vi "Autonomous Independent.vi"() -> ()   [LabVIEW 2018]
doc: "This VI is called when autonomous begins, and will automatically be terminated when autonomous ends. You can carry out timed or sensor driven robot movement independently without needing to return to the caller."
uses:
  <vilib>/Rock Robotics/WPI/ThirdParty/Phoenix-LabVIEW/Motor Controller/Controls/CTRE_Phoenix_MotorControl_ControlMode.ctl
  <vilib>/Rock Robotics/WPI/Utilities/WPI_GetSetVariantRefNum.vi
  <vilib>/Rock Robotics/Network Tables/NT Read String.vi
  <vilib>/Rock Robotics/Network Tables/NT Write Numeric Array.vi
  <vilib>/Rock Robotics/WPI/ThirdParty/Phoenix-LabVIEW/Motor Controller/Get/CTRE_Phoenix_MotorController_GetOutputCurrent_Enhanced.vi
  <vilib>/Rock Robotics/WPI/ThirdParty/Phoenix-LabVIEW/Motor Controller/Get/CTRE_Phoenix_MotorController_GetSelectedSensorData.vi
  <vilib>/Rock Robotics/WPI/RobotDrive/WPI_RobotDriveArcadeDrive_Standard(NoSaturation).vi
panel:
  out "Current Left":T1(graph)
  out "Current Right":T1(graph)
  out "Velocity":T2(graph)
  out "Position":T3(graph)
  in  "Speed %":dbl=0.4
  in  "Array of robot movements":T4(array[cluster])=[{"X Joystick Value"=0.39393939393939403, "Y Joystick Value"=0.0, "Delay (sec)"=1.0, "Movement Name"="turn"}, {"X Joystick Value"=-0.3737373737373737, "Y Joystick Value"=0.0, "Delay (sec)"=1.0, "Movement Name"="turn back"}] {"Y Joystick Value" scale=1.0..-1.0; "X Joystick Value" scale=-1.0..1.0}
  # "Be sure to right-click and choose Data Operations>>Make Current Value default if you want to save the array values with the VI"
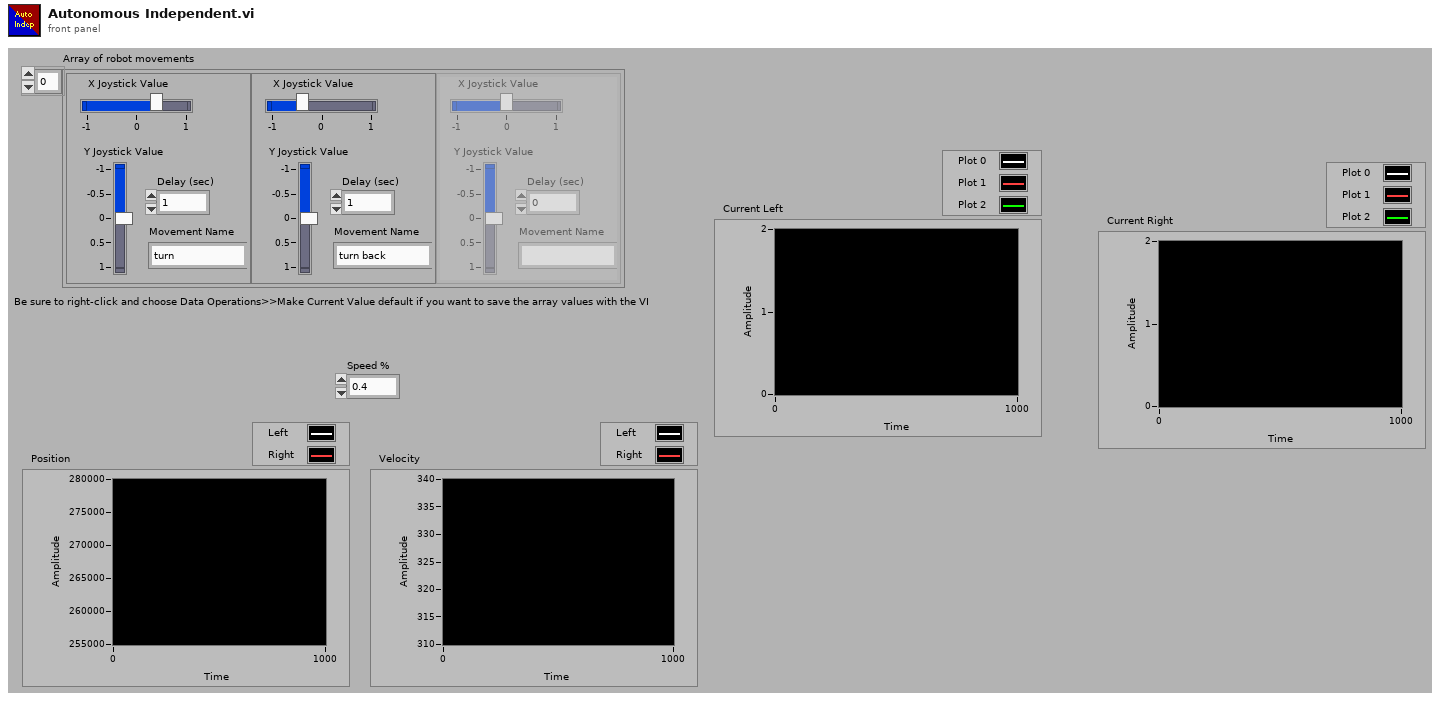
[diagram p1: front panel]
types:
  T1 = cluster{"Output Current":dbl, "Output Current":dbl, "Output Current":dbl}
  T2 = cluster{"Velocity (Raw Sensor Units per 100 ms)":i32, "Velocity (Raw Sensor Units per 100 ms)":i32}
  T3 = cluster{"Position (Raw Sensor Units)":i32, "Position (Raw Sensor Units)":i32}
  T4 = cluster{"X Joystick Value":dbl, "Y Joystick Value":dbl, "Delay (sec)":dbl, "Movement Name":string}[]
  T5 = typedef "WPI_JoystickDevRef.ctl" = cluster{"Device":T6}
  T6 = typedef "WPI_JoystickDeviceEnum.ctl" = enum16{"USB 0", "USB 1", "USB 2", "USB 3", "USB 4", "USB 5"}
  T7 = typedef "WPI_MotorControlDeviceRef.ctl" = cluster{"DeviceStatus":errorcluster, "Type":T8, "PWM":cluster{"PWM Channel":T9, "DeadBand":T10}, "CAN":cluster{"Device Number":u8, "SetOutput VI Ref":variant, "GetOutput VI Ref":variant, "Enable VI Ref":variant, "Disable VI Ref":variant, "Data":variant}, "Invert":bool, "DIO PWM":cluster{"PWM \"Enable\" Channel":T9, "DIOChannel":T11, "PWM Rate":dbl}}
  T8 = typedef "WPI_MotorControlType.ctl" = enum16{"PWM", "CAN", "DIO PWM"}
  T9 = typedef "FPGA_DIOPWMChannel.ctl" = enum8{"PWM 0", "PWM 1", "PWM 2", "PWM 3", "PWM 4", "PWM 5", "PWM 6", "PWM 7", "PWM 8", "PWM 9", "PWM MXP 0", "PWM MXP 1", "PWM MXP 2", "PWM MXP 3", "PWM MXP 4", "PWM MXP 5", "PWM MXP 6", "PWM MXP 7", "PWM MXP 8", "PWM MXP 9", "Invalid"}
  T10 = typedef "WPI_PWMDeadband.ctl" = cluster{"Name":string, "maxPositivePwm":i32, "minPositivePwm":i32, "centerPwm":i32, "maxNegativePwm":i32, "minNegativePwm":i32, "angularRange":u16}
  T11 = typedef "FPGA_DIOChannel.ctl" = enum8{"DIO 0", "DIO 1", "DIO 2", "DIO 3", "DIO 4", "DIO 5", "DIO 6", "DIO 7", "DIO 8", "DIO 9", "DIO MXP 0", "DIO MXP 1", "DIO MXP 2", "DIO MXP 3", "DIO MXP 4", "DIO MXP 5", "DIO MXP 6", "DIO MXP 7", "DIO MXP 8", "DIO MXP 9", "DIO MXP 10", "DIO MXP 11", "DIO MXP 12", "DIO MXP 13", "DIO MXP 14", "DIO MXP 15", "SPI Port CS1", "SPI Port CS2", "SPI Port CS3", "SPI Port MISO", "SPI Port MOSI", "Invalid"}
  T12 = typedef "CTRE_Phoenix_MotorControl_ControlMode.ctl" = u16
  T13 = typedef "WPI_RobotDriveDevRef.ctl" = cluster{"DevStatus":errorcluster, "Motors[]":T7[], "Square Inputs":bool, "Max Output":dbl}
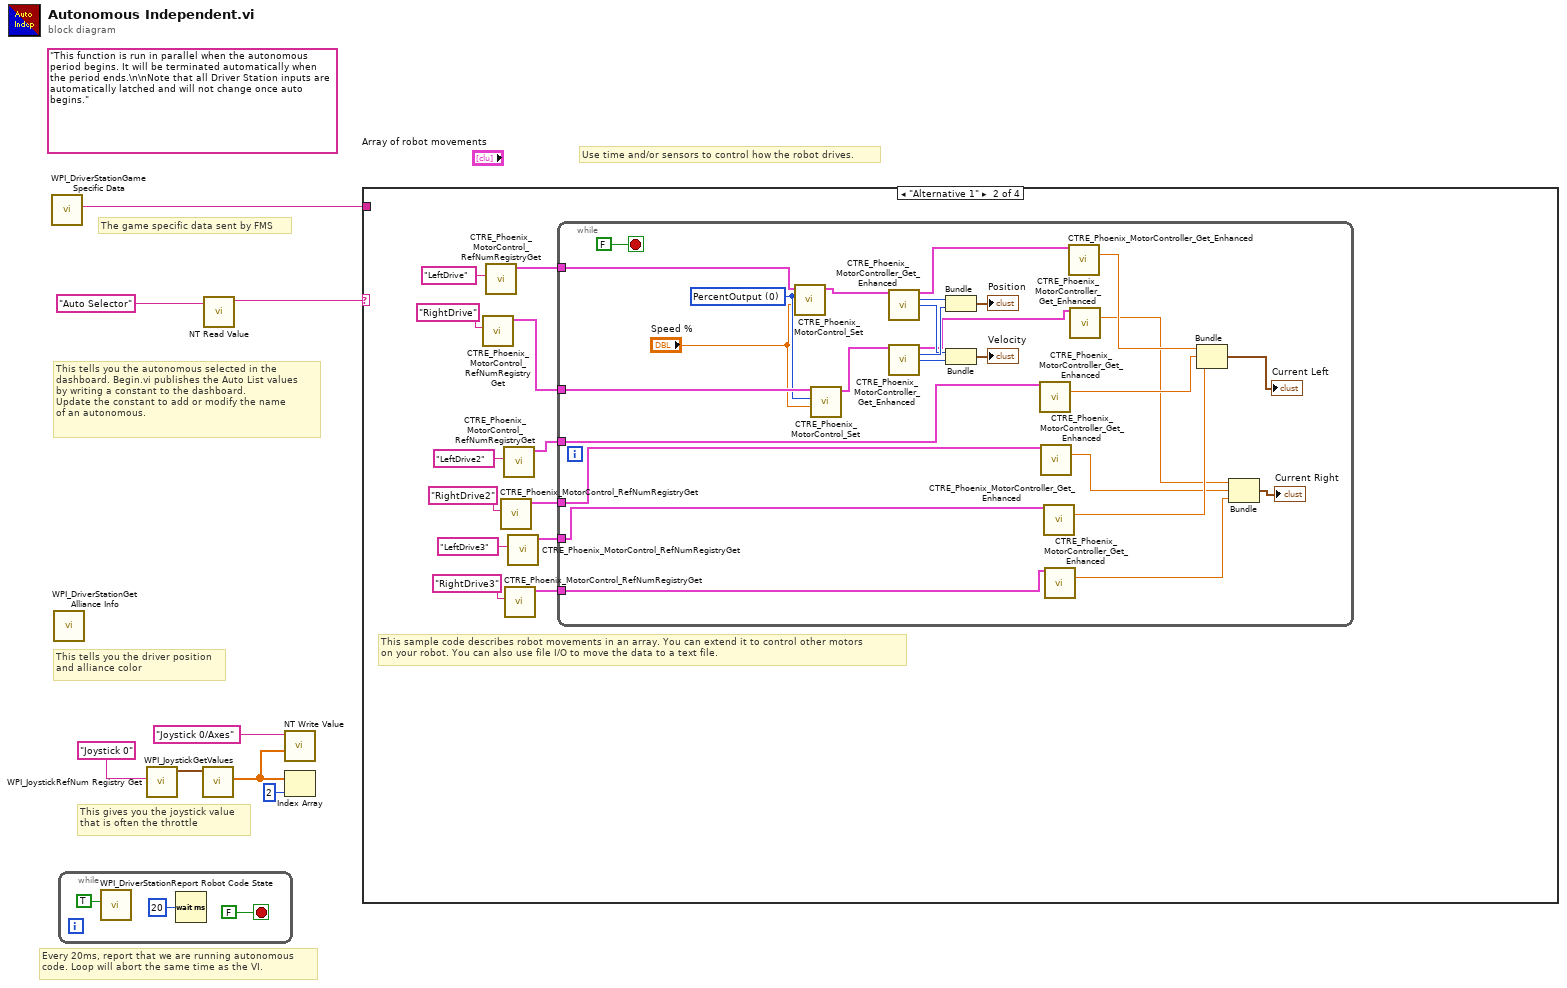
[diagram p0: block diagram]
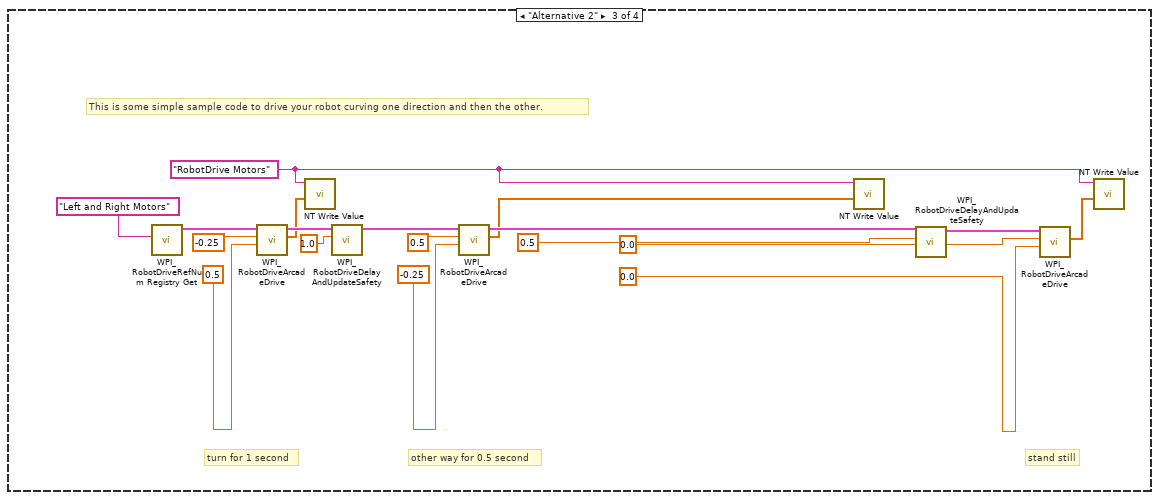
[diagram p3: hidden frame]
diagram:
  (unwired) "This function is run in parallel when the autonomous period begins. It will be terminated automatically when the period ends.\n\nNote that all Driver Station inputs are automatically latched and will not change once auto begins."
  # "The game specific data sent by FMS"
  # "This tells you the autonomous selected in the \ndashboard. Begin.vi publishes the Auto List values\nby writing a constant to the dashboard.\nUpdate the constant to add or modify the name\nof an autonomous."
  # "Every 20ms, report that we are running autonomous\ncode. Loop will abort the same time as the VI."
  # "This gives you the joystick value\nthat is often the throttle"
  # "Use time and/or sensors to control how the robot drives."
  # "This tells you the driver position\nand alliance color"
  n1 = call <vilib>:"WPI_DriverStationGame Specific Data.vi"() -> ("Game Specific Data"=w1:string)  [unwired: 11 in]
  n2 = call <vilib>:"WPI_DriverStationGet Alliance Info.vi"() -> ()  [unwired: 12 out]
  n3 = while {
    stop <- FALSE stop-if-true
    n4 = call <vilib>:"WPI_DriverStationReport Robot Code State.vi"("Autonomous"=TRUE) -> ()  [unwired: 10 in, 1 out]
    n5 = Wait (ms)(milliseconds to wait=u32 20) -> ()  [unwired: 1 out]
  }
  n6 = call <vilib>:"WPI_JoystickRefNum Registry Get.vi"("refnum name"="Joystick 0") -> ("JoystickDevRef"=w7:T5)  [unwired: 1 in, 9 out]
  n7 = call <vilib>:"WPI_JoystickGetValues.vi"("JoystickDevRef"=w7) -> ("Axes"=w3:dbl[])  [unwired: 6 in, 4 out]
  n8 = call-poly <vilib>:"NT Read Value.vi"("Name"="Auto Selector") -> ("String"=w4:string)  [unwired: 9 in, 1 out]
  n9 = call-poly <vilib>:"NT Write Value.vi"("Numeric Array"=w3, "Name"="Joystick 0/Axes") -> ()  [unwired: 9 in, 1 out]
  n10 = Index Array(array=w3, index=2) -> ()  [unwired: 1 out]
  n11 = case shown="\"Alternative 1\"" w4 {
    tunnel: w1 -> [_ _ _ _]
    frame Default {
      # "You can put your main auto here, or you can right-click on the case and make any\nother frame be the default case."
      # "This is the frame that will execute if no selection is made, or if it is not recognized"
    }
    frame "Alternative 1" {
      # "This sample code describes robot movements in an array. You can extend it to control other motors\non your robot. You can also use file I/O to move the data to a text file."
      n12 = call <vilib>:"CTRE_Phoenix_MotorControl_RefNumRegistryGet.vi"("refnum name"="RightDrive") -> ("PhoenixMotorControlDevRef"=w20:T7)  [unwired: 9 in, 1 out]
      n13 = call <vilib>:"CTRE_Phoenix_MotorControl_RefNumRegistryGet.vi"("refnum name"="LeftDrive") -> ("PhoenixMotorControlDevRef"=w21:T7)  [unwired: 9 in, 1 out]
      n14 = call <vilib>:"CTRE_Phoenix_MotorControl_RefNumRegistryGet.vi"("refnum name"="RightDrive2") -> ("PhoenixMotorControlDevRef"=w14:T7)  [unwired: 9 in, 1 out]
      n15 = call <vilib>:"CTRE_Phoenix_MotorControl_RefNumRegistryGet.vi"("refnum name"="LeftDrive2") -> ("PhoenixMotorControlDevRef"=w15:T7)  [unwired: 9 in, 1 out]
      n16 = call <vilib>:"CTRE_Phoenix_MotorControl_RefNumRegistryGet.vi"("refnum name"="RightDrive3") -> ("PhoenixMotorControlDevRef"=w12:T7)  [unwired: 9 in, 1 out]
      n17 = call <vilib>:"CTRE_Phoenix_MotorControl_RefNumRegistryGet.vi"("refnum name"="LeftDrive3") -> ("PhoenixMotorControlDevRef"=w13:T7)  [unwired: 9 in, 1 out]
      n18 = while {
        tunnel: w21 -> [w50]
        tunnel: w20 -> [w49]
        tunnel: w15 -> [w35]
        tunnel: w14 -> [w34]
        tunnel: w13 -> [w33]
        tunnel: w12 -> [w32]
        stop <- FALSE stop-if-true
        w48 = T12 0 items=["PercentOutput"=0, "Position"=1, "Velocity"=2, "Current"=3, "Follower"=5, "MotionProfile"=6, "MotionMagic"=7, "MotionProfileArc"=10, "Disabled"=15] ("Control Mode")
        n19 = call <vilib>:"CTRE_Phoenix_MotorControl_Set.vi"("Output"="Speed %", "Control Mode"=w48, "PhoenixMotorControlDevRef"=w50) -> ("PhoenixMotorControlDevRef"=w45:T7)  [unwired: 7 in, 1 out]
        n20 = call <vilib>:"CTRE_Phoenix_MotorControl_Set.vi"("Output"="Speed %", "Control Mode"=w48, "PhoenixMotorControlDevRef"=w49) -> ("PhoenixMotorControlDevRef"=w44:T7)  [unwired: 7 in, 1 out]
        n21 = call-poly <vilib>:"CTRE_Phoenix_MotorController_Get_Enhanced.vi"("PhoenixMotorControlDevRef"=w45) -> ("PhoenixMotorControlDevRef"=w37:T7, "Position (Raw Sensor Units)"=w41:i32, "Velocity (Raw Sensor Units per 100 ms)"=w40:i32)  [unwired: 11 in, 1 out]
        n22 = call-poly <vilib>:"CTRE_Phoenix_MotorController_Get_Enhanced.vi"("PhoenixMotorControlDevRef"=w44) -> ("PhoenixMotorControlDevRef"=w36:T7, "Position (Raw Sensor Units)"=w42:i32, "Velocity (Raw Sensor Units per 100 ms)"=w39:i32)  [unwired: 11 in, 1 out]
        n23 = Bundle("Position (Raw Sensor Units)"=w41, "Position (Raw Sensor Units)"=w42) -> (→"Position":T3)  [unwired: 1 in]
        n24 = Bundle("Velocity (Raw Sensor Units per 100 ms)"=w40, "Velocity (Raw Sensor Units per 100 ms)"=w39) -> (→"Velocity":T2)  [unwired: 1 in]
        n25 = call-poly <vilib>:"CTRE_Phoenix_MotorController_Get_Enhanced.vi"("PhoenixMotorControlDevRef"=w35) -> ("Output Current"=w30:dbl)  [unwired: 12 in, 2 out]
        n26 = call-poly <vilib>:"CTRE_Phoenix_MotorController_Get_Enhanced.vi"("PhoenixMotorControlDevRef"=w34) -> ("Output Current"=w27:dbl)  [unwired: 12 in, 2 out]
        n27 = call-poly <vilib>:"CTRE_Phoenix_MotorController_Get_Enhanced.vi"("PhoenixMotorControlDevRef"=w33) -> ("Output Current"=w29:dbl)  [unwired: 12 in, 2 out]
        n28 = call-poly <vilib>:"CTRE_Phoenix_MotorController_Get_Enhanced.vi"("PhoenixMotorControlDevRef"=w32) -> ("Output Current"=w26:dbl)  [unwired: 12 in, 2 out]
        n29 = call-poly <vilib>:"CTRE_Phoenix_MotorController_Get_Enhanced.vi"("PhoenixMotorControlDevRef"=w37) -> ("Output Current"=w31:dbl)  [unwired: 12 in, 2 out]
        n30 = call-poly <vilib>:"CTRE_Phoenix_MotorController_Get_Enhanced.vi"("PhoenixMotorControlDevRef"=w36) -> ("Output Current"=w28:dbl)  [unwired: 12 in, 2 out]
        n31 = Bundle("Output Current"=w31, "Output Current"=w30, "Output Current"=w29) -> (→"Current Left":T1)  [unwired: 1 in]
        n32 = Bundle("Output Current"=w28, "Output Current"=w27, "Output Current"=w26) -> (→"Current Right":T1)  [unwired: 1 in]
      }
    }
    frame "Alternative 2" {
      w52 = "RobotDrive Motors" ("Name")
      # "This is some simple sample code to drive your robot curving one direction and then the other."
      # "stand still"
      # "other way for 0.5 second"
      # "turn for 1 second"
      n33 = call <vilib>:"WPI_RobotDriveRefNum Registry Get.vi"("refnum name"="Left and Right Motors") -> ("RobotDriveDevRef"=w68:T13)  [unwired: 1 in, 9 out]
      n34 = call-poly <vilib>:"WPI_RobotDriveArcadeDrive.vi"("Y axis value"=0.5 ("X axis value"), "X axis value"=-0.25, "RobotDriveDevRef"=w68) -> ("Motor Values"=w51:dbl[], "RobotDriveDevRef"=w61:T13)  [unwired: 1 in, 6 out]
      n35 = call-poly <vilib>:"NT Write Value.vi"("Numeric Array"=w51, "Name"=w52) -> ()  [unwired: 9 in, 1 out]
      n36 = call <vilib>:"WPI_RobotDriveDelayAndUpdateSafety.vi"("Delay (s)"=1.0, "RobotDriveDevRef"=w61) -> ("RobotDriveDevRef 2"=w62:T13)  [unwired: 8 in, 1 out]
      n37 = call-poly <vilib>:"WPI_RobotDriveArcadeDrive.vi"("Y axis value"=-0.25 ("X axis value"), "X axis value"=0.5, "RobotDriveDevRef"=w62) -> ("Motor Values"=w53:dbl[], "RobotDriveDevRef"=w63:T13)  [unwired: 1 in, 6 out]
      n38 = call-poly <vilib>:"NT Write Value.vi"("Numeric Array"=w53, "Name"=w52) -> ()  [unwired: 9 in, 1 out]
      n39 = call <vilib>:"WPI_RobotDriveDelayAndUpdateSafety.vi"("Delay (s)"=0.5, "RobotDriveDevRef"=w63) -> ("RobotDriveDevRef 2"=w64:T13)  [unwired: 8 in, 1 out]
      n40 = call-poly <vilib>:"WPI_RobotDriveArcadeDrive.vi"("Y axis value"=0.0 ("X axis value"), "X axis value"=0.0, "RobotDriveDevRef"=w64) -> ("Motor Values"=w54:dbl[])  [unwired: 1 in, 7 out]
      n41 = call-poly <vilib>:"NT Write Value.vi"("Numeric Array"=w54, "Name"=w52) -> ()  [unwired: 9 in, 1 out]
    }
    frame "Your Turn" {
    }
  }
